vi "Enqueue Frame.vi"(8 "error in":errorcluster, 11 "Data":string[][](array[string])) -> (0 "error out":errorcluster, 3 "overflow?":bool)   [LabVIEW 2025, in "Automotive Ethernet Bus Monitor.lvclass"]
doc: "Add a frame to the buffer queue."
uses:
  Automotive Ethernet Bus Monitor.lvclass
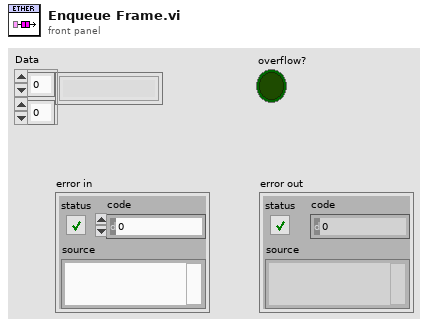
[diagram p1: front panel]
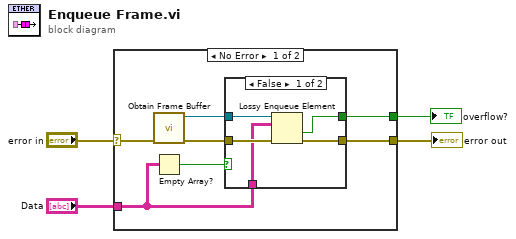
[diagram p0: block diagram]
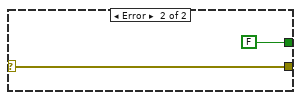
[diagram p3: hidden frame]
diagram:
  n1 = case shown="No Error" "error in" {
    selector: "error in" -> [w11 w19]
    tunnel: [w9 w19] -> w3
    tunnel: "Data" -> [w6 _]
    tunnel: [w7 FALSE ("overflow?")] -> w1
    frame No Error {
      n2 = call "Obtain Frame Buffer.vi"("error in"=w11) -> ("error out"=w10:errorcluster, "queue out"=w8:refnum<queue>)  [unwired: 9 in]
      n3 = Empty Array?(array=w6) -> (empty?=w5:bool)
      n4 = case shown="False" w5 {
        tunnel: w10 -> [w16 w17]
        tunnel: [w15 w17] -> w9
        tunnel: w8 -> [w14 _]
        tunnel: w6 -> [w13 _]
        tunnel: [w12 _] -> w7
        frame False {
          n5 = Lossy Enqueue Element(queue=w14, element=w13, error in (no error)=w16) -> (overflow?=w12:bool, error out=w15:errorcluster)  [unwired: 2 out]
        }
        frame True {
        }
      }
    }
    frame Error {
    }
  }
  "error out" <- w3
  "overflow?" <- w1
